vi "VI Grader.vi"(8 "Error In":errorcluster, 10 "Challenge Config":T4, 11 "VIChallenge Config":T5={"AWS Credentials"={"AWSAccessKeyId"="", "Secret Key"=""}, "AWS Account Number"="", "SQS Jobs"=refnum, "SQS Status"=refnum, "Source Dir"=path "", "Working Dir"=path "", "Output Dir"=path "", "Archive Dir"=path "", "job"={"job_id"="", "challenge_id"="", "user_id"="", "s3_source_bucket"="", "s3_source_directory"="", "s3_source_filename"="", "status_queue_name"="", "username"=""}, "Database Ref"=refnum, "Challenge Dir"=path "", "Challenges"=[]}) -> (0 "Error Out":errorcluster, 2 "Grader Result":T1={"Id"="", "Score"={"Status"=enum."Passed", "cpu_time"=0, "max_memory"=0, "style_score"=0, "score0"="", "score1"="", "score2"="", "score3"="", "score4"="", "score5"=""}}, 3 "VIChallenge Config":T5)   [LabVIEW 2013, in "VIChallenge.lvlib"]
uses:
  <vilib>/LabVIEW Hacker/VIChallenge/VIChallenge.lvlib
  <vilib>/LabVIEW Hacker/VIChallenge/Private/Type Defs/VIChallenge Config.ctl
  <vilib>/National Instruments/NI Amazon Web Services (AWS) Toolkit for LabVIEW/SQS/VI Source/AWS SQS Class/AWS_SQS.lvclass
  <vilib>/National Instruments/NI Amazon Web Services (AWS) Toolkit for LabVIEW/AWS Core Lib/VI Source/Canonicals/AWS_Core Canonical Credentials/Canonical Credentials.lvclass
  <vilib>/National Instruments/NI Amazon Web Services (AWS) Toolkit for LabVIEW/AWS Core Lib/VI Source/Canonicals/AWS_Core Canonical Required Parameters/Canonical Required Parameters.lvclass
  <vilib>/National Instruments/NI Amazon Web Services (AWS) Toolkit for LabVIEW/SQS/VI Source/Canonicals/Canonical CreateQueue/Canonical CreateQueue.lvclass
  <vilib>/National Instruments/NI Amazon Web Services (AWS) Toolkit for LabVIEW/SQS/VI Source/Canonicals/Canonical ListQueues/Canonical ListQueues.lvclass
  <vilib>/National Instruments/NI Amazon Web Services (AWS) Toolkit for LabVIEW/SQS/VI Source/Canonicals/Canonical AddPermission/Canonical AddPermission.lvclass
  <vilib>/National Instruments/NI Amazon Web Services (AWS) Toolkit for LabVIEW/SQS/VI Source/Canonicals/Canonical ChangeMessageVisibility/Canonical ChangeMessageVisibility.lvclass
  <vilib>/National Instruments/NI Amazon Web Services (AWS) Toolkit for LabVIEW/SQS/VI Source/Canonicals/Canonical ChangeMessageVisibilityBatch/Canonical ChangeMessageVisibilityBatch.lvclass
  <vilib>/National Instruments/NI Amazon Web Services (AWS) Toolkit for LabVIEW/SQS/VI Source/Canonicals/Canonical DeleteMessage/Canonical DeleteMessage.lvclass
  <vilib>/National Instruments/NI Amazon Web Services (AWS) Toolkit for LabVIEW/SQS/VI Source/Canonicals/Canonical DeleteMessageBatch/Canonical DeleteMessageBatch.lvclass
  <vilib>/National Instruments/NI Amazon Web Services (AWS) Toolkit for LabVIEW/SQS/VI Source/Canonicals/Canonical GetQueueAttributes/Canonical GetQueueAttributes.lvclass
  <vilib>/National Instruments/NI Amazon Web Services (AWS) Toolkit for LabVIEW/SQS/VI Source/Canonicals/Canonical GetQueueUrl/Canonical GetQueueUrl.lvclass
  <vilib>/National Instruments/NI Amazon Web Services (AWS) Toolkit for LabVIEW/SQS/VI Source/Canonicals/Canonical ReceiveMessage/Canonical ReceiveMessage.lvclass
  <vilib>/National Instruments/NI Amazon Web Services (AWS) Toolkit for LabVIEW/SQS/VI Source/Canonicals/Canonical RemovePermission/Canonical RemovePermission.lvclass
  <vilib>/National Instruments/NI Amazon Web Services (AWS) Toolkit for LabVIEW/SQS/VI Source/Canonicals/Canonical SendMessage/Canonical SendMessage.lvclass
  <vilib>/National Instruments/NI Amazon Web Services (AWS) Toolkit for LabVIEW/SQS/VI Source/Canonicals/Canonical SendMessageBatch/Canonical SendMessageBatch.lvclass
  <vilib>/National Instruments/NI Amazon Web Services (AWS) Toolkit for LabVIEW/SQS/VI Source/Canonicals/Canonical SetQueueAttributes/Canonical SetQueueAttributes.lvclass
  <vilib>/National Instruments/NI Amazon Web Services (AWS) Toolkit for LabVIEW/AWS Core Lib/VI Source/Typedefs/AWS_AWS Credentials.ctl
  <vilib>/LabVIEW Hacker/VIChallenge/Private/Type Defs/JSON_job.ctl
  <vilib>/addons/database/Connection.llb/Conn ObjectReference.ctl
  <vilib>/LabVIEW Hacker/VIChallenge/Private/Grader/Type Defs/Challenge.ctl
  <vilib>/LabVIEW Hacker/VIChallenge/Private/Grader/Type Defs/Grader Result.ctl
  <vilib>/LabVIEW Hacker/VIChallenge/Private/Type Defs/Database/Score.ctl
  <vilib>/LabVIEW Hacker/VIChallenge/Private/Grader/Type Defs/UTF Status.ctl
  <vilib>/National Instruments/NI Amazon Web Services (AWS) Toolkit for LabVIEW/AWS Core Lib/VI Source/AWS_Core.lvlib
  <vilib>/addons/database/NI_Database_API.lvlib
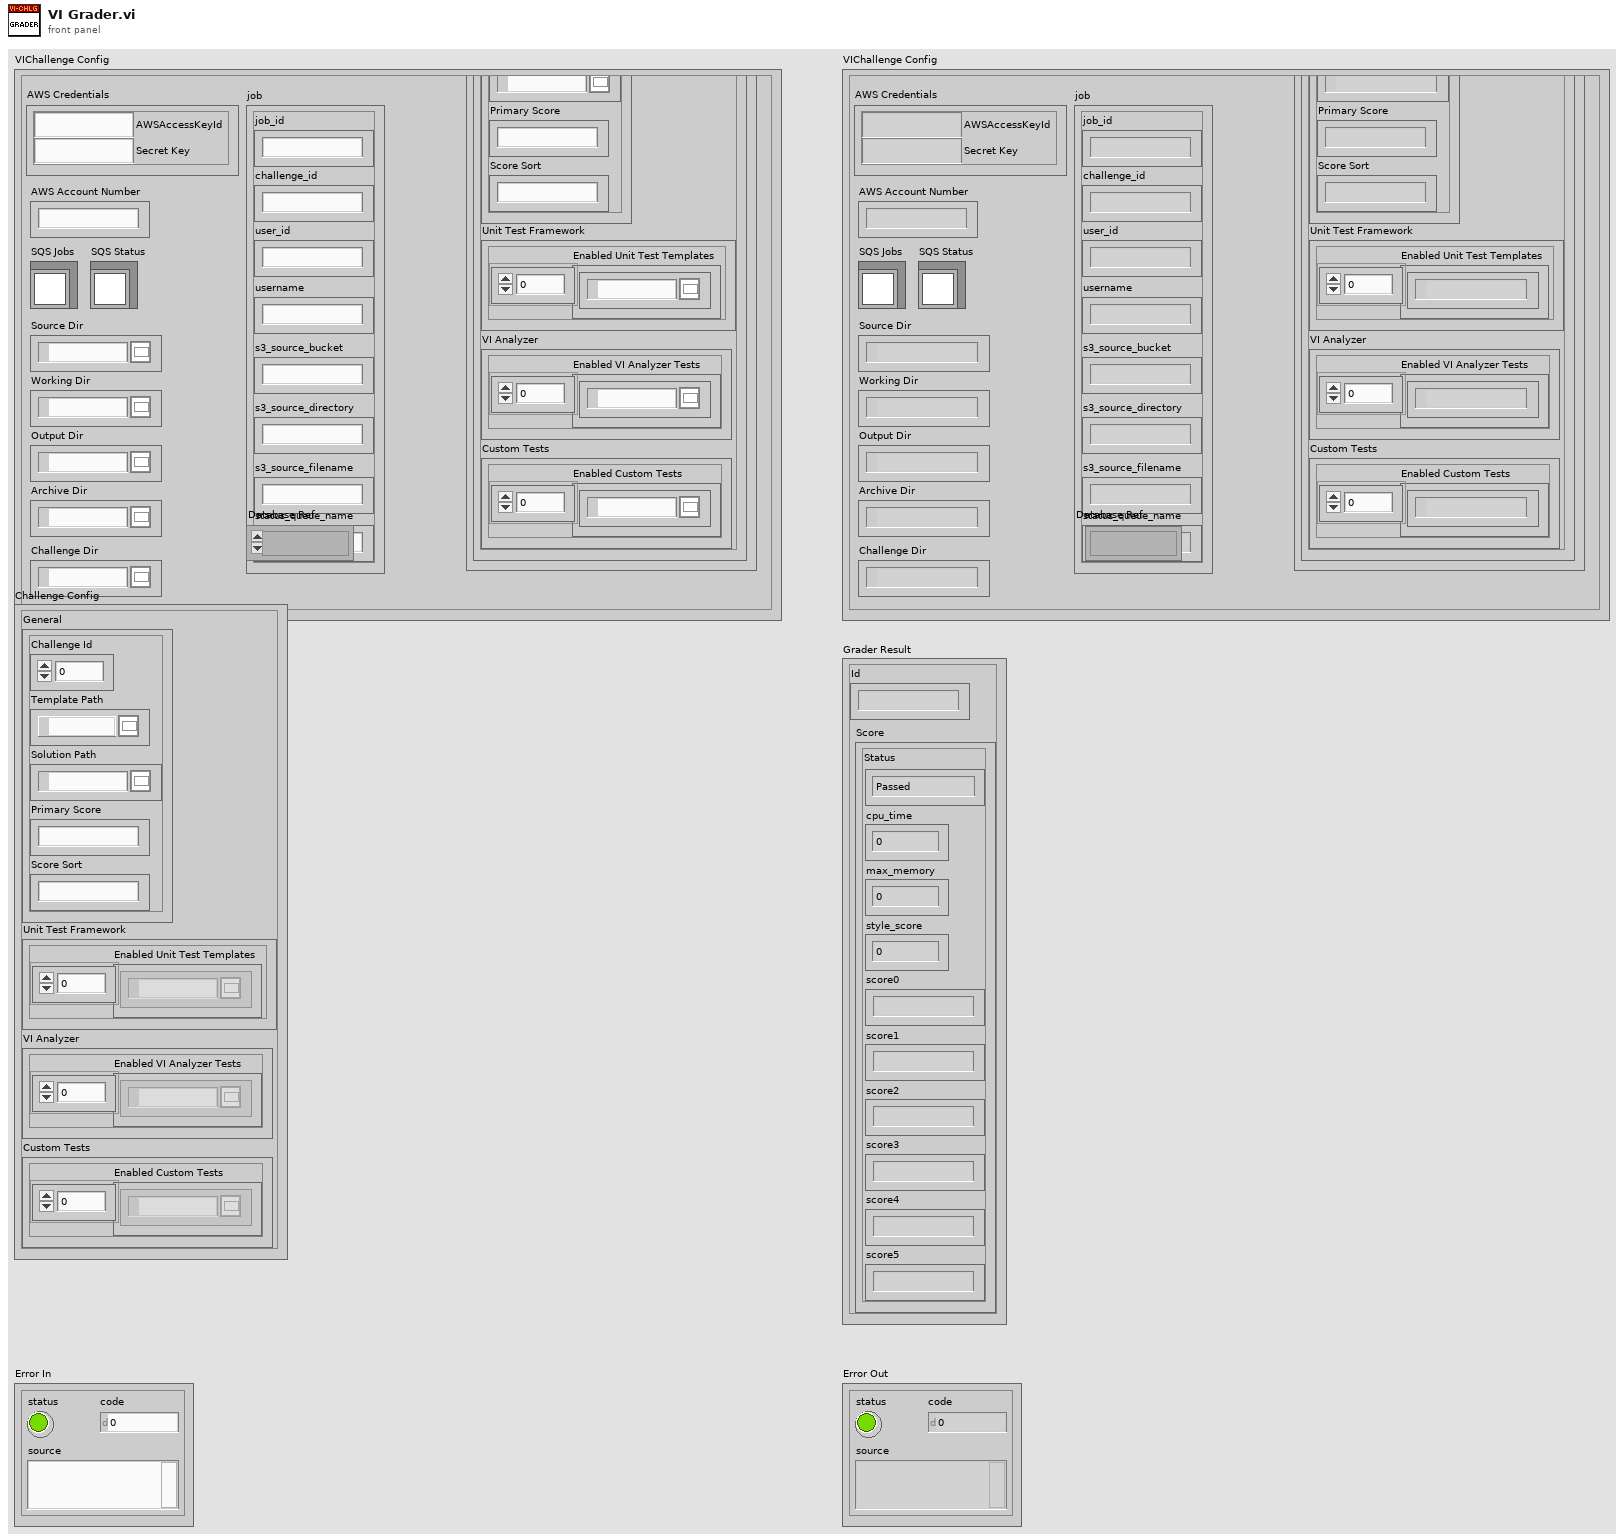
[diagram p1: front panel]
types:
  T1 = typedef "VIChallenge.lvlib/Grader Result.ctl" = cluster{"Id":string, "Score":T2}
  T2 = typedef "VIChallenge.lvlib/Score.ctl" = cluster{"Status":T3, "cpu_time":i32, "max_memory":i32, "style_score":i32, "score0":string, "score1":string, "score2":string, "score3":string, "score4":string, "score5":string}
  T3 = typedef "VIChallenge.lvlib/UTF Status.ctl" = enum16{"Null", "Passed", "Failed", "Error", "Skipped", "Not Processed"}
  T4 = typedef "VIChallenge.lvlib/Challenge.ctl" = cluster{"General":cluster{"Challenge Id":i32, "Template Path":path, "Solution Path":path, "Primary Score":string, "Score Sort":string}, "Unit Test Framework":cluster{"Enabled Unit Test Templates":path[]}, "VI Analyzer":cluster{"Enabled VI Analyzer Tests":path[]}, "Custom Tests":cluster{"Enabled Custom Tests":path[]}}
  T5 = typedef "VIChallenge.lvlib/VIChallenge Config.ctl" = cluster{"AWS Credentials":T6, "AWS Account Number":string, "SQS Jobs":refnum<class "AWS_SQS.lvclass">, "SQS Status":refnum<class "AWS_SQS.lvclass">, "Source Dir":path, "Working Dir":path, "Output Dir":path, "Archive Dir":path, "job":T7, "Database Ref":T8, "Challenge Dir":path, "Challenges":T4[]}
  T6 = typedef "AWS_Core.lvlib/AWS_AWS Credentials.ctl" = cluster{"AWSAccessKeyId":string, "Secret Key":string}
  T7 = typedef "VIChallenge.lvlib/JSON_job.ctl" = cluster{"job_id":string, "challenge_id":string, "user_id":string, "s3_source_bucket":string, "s3_source_directory":string, "s3_source_filename":string, "status_queue_name":string, "username":string}
  T8 = typedef "NI_Database_API.lvlib/Conn ObjectReference.ctl" = refnum<k1>
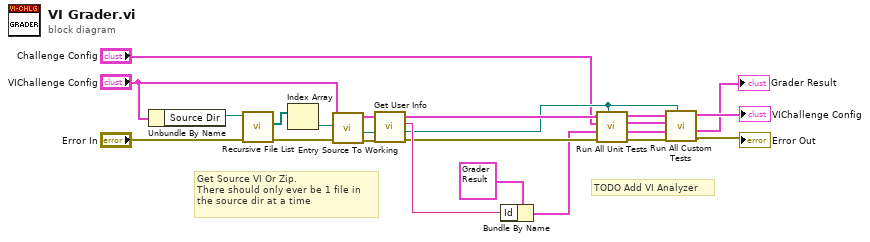
[diagram p0: block diagram]
diagram:
  # "TODO Add VI Analyzer"
  # "Get Source VI Or Zip.\nThere should only ever be 1 file in \nthe source dir at a time"
  n1 = Unbundle By Name("VIChallenge Config") -> ("Source Dir"=w17:path)
  n2 = call <vilib>:"Recursive File List.vi"("error in (no error)"="Error In", "Folder Path"=w17) -> ("error out"=w15:errorcluster, "All Files in Dir"=w14:path[])  [unwired: 5 in, 3 out]
  n3 = Index Array(array=w14) -> (element=w13:path)  [unwired: 1 in]
  n4 = call <vilib>:"Entry Source To Working.vi"("Error In"=w15, "Source File"=w13, "VIChallenge Config"="VIChallenge Config") -> ("Error Out"=w20:errorcluster, "Main VI Path"=w21:path, "VIChallenge Config"=w22:T5)  [unwired: 6 in]
  n5 = call <vilib>:"Get User Info.vi"("Error In"=w20, "Main VI"=w21, "VIChallenge Config"=w22) -> ("Error Out"=w5:errorcluster, "Dup Main VI"=w4:path, "User Id"=w18:string, "VIChallenge Config"=w8:T5)  [unwired: 5 in]
  n6 = Bundle By Name(cluster=T1 {"Id"="", "Score"={"Status"=enum."Null", "cpu_time"=-1, "max_memory"=-1, "style_score"=-1, "score0"="", "score1"="", "score2"="", "score3"="", "score4"="", "score5"=""}} ("Grader Result"), "Id"=w18) -> (w2:T1)
  n7 = call <vilib>:"Run All Unit Tests.vi"("Main VI"=w4, "Error In"=w5, "Grader Result in"=w2, "Challenge Config"="Challenge Config", "VIChallenge Config"=w8) -> ("Error Out"=w12:errorcluster, "Grader Result"=w9:T1, "Challenge Config"=w10:T4, "VIChallenge Config"=w11:T5)  [unwired: 3 in]
  n8 = call <vilib>:"Run All Custom Tests.vi"("Main VI"=w4, "Error In"=w12, "Grader Result in"=w9, "Challenge Config"=w10, "VIChallenge Config"=w11) -> ("Error Out"=→"Error Out":errorcluster, "Grader Result"=→"Grader Result":T1, "VIChallenge Config"=→"VIChallenge Config":T5)  [unwired: 3 in, 1 out]
